vi "SetGum Machine.lvclass.vi"(8 "error in (no error)":errorcluster, 10 "Gum Machine.lvclass":refnum<class "Gum Machine.lvclass">, 11 "reference in":refnum<class "Has Coin State.lvclass">) -> (0 "error out":errorcluster, 3 "reference out":refnum<class "Has Coin State.lvclass">)   [LabVIEW 2013, in "Has Coin State.lvclass"]
uses:
  Has Coin State.lvclass
  Gum Machine_class/Gum Machine.lvclass
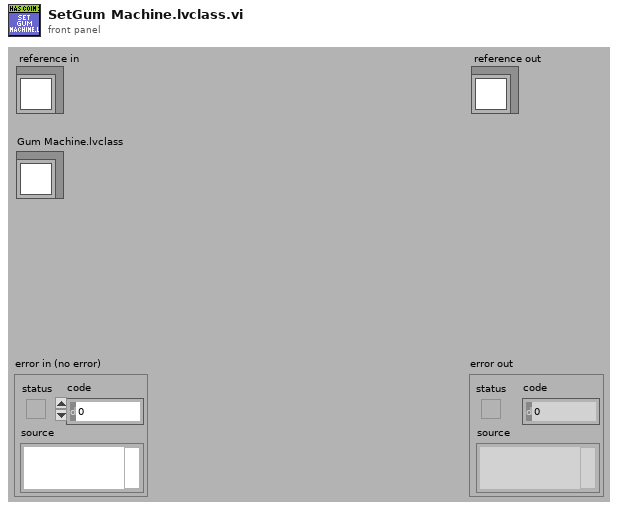
[diagram p1: front panel]
types:
  T1 = typedef "Has Coin State.lvclass/ObjectAttributesRef.ctl" = refnum<data-value>
  T2 = typedef "Has Coin State.lvclass/ObjectAttributes.ctl" = cluster{"Gum Machine.lvclass":refnum<class "Gum Machine.lvclass">}
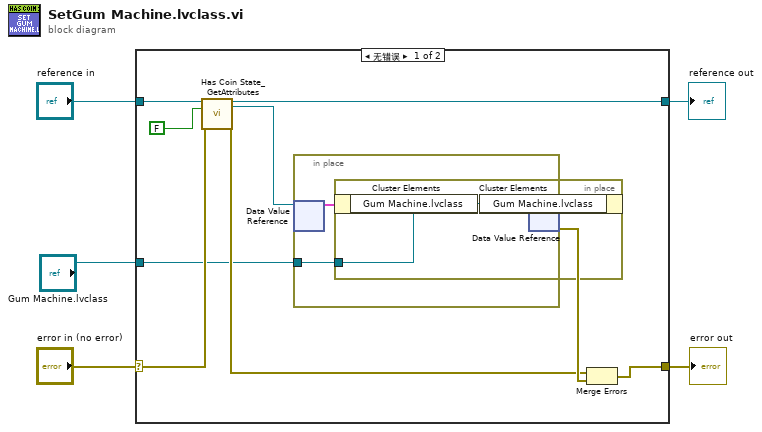
[diagram p0: block diagram]
diagram:
  n1 = case shown="无错误" "error in (no error)" {
    selector: "error in (no error)" -> [w14 w20]
    tunnel: [w8 w20] -> w4
    tunnel: [w13 w19] -> w2
    tunnel: "reference in" -> [w12 w19]
    tunnel: "Gum Machine.lvclass" -> [w6 _]
    frame No Error {
      n2 = call "Has Coin State_GetAttributes.vi"("reference in"=w12, "return data? (T)"=FALSE, "error in (no error)"=w14) -> ("reference out"=w13:refnum<class "Has Coin State.lvclass">, "attributes ref"=w7:T1, "error out"=w9:errorcluster)  [unwired: 13 in, 1 out]
      n3 = in-place {
        in-place-border: w6 -> [w15]
        n4 = in-place-dvr #1(w7) -> (w16:T2)  [unwired: 1 out]
        n5 = in-place {
          in-place-border: w15 -> [w18]
          n6 = in-place-cluster #2(w16) -> ()  [unwired: 1 out]
          n7 = in-place-cluster #2("Gum Machine.lvclass"=w18) -> (w17:T2)
        }
        n8 = in-place-dvr #1(w17) -> (w10:errorcluster)  [unwired: 1 out]
      }
      n9 = Merge Errors(w9, w10) -> (w8:errorcluster)
    }
    frame Error {
    }
  }
  "error out" <- w4
  "reference out" <- w2
